vi "CheckImageQuality.vi"(8 "error in (no error)":errorcluster, 11 "Image":T1) -> (0 "error out":errorcluster, 1 "Standard  Variation":sgl, 2 "Mean Value":sgl, 3 "Within Range":bool, 5 "Range":sgl)   [LabVIEW 2017]
uses:
  <vilib>/vision/Image Controls.llb/IMAQ Image.ctl
  <vilib>/vision/NI_Vision_Development_Module.lvlib
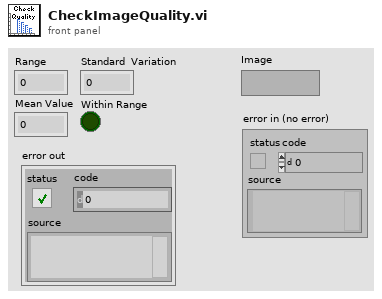
[diagram p1: front panel]
types:
  T1 = typedef "IMAQ Image.ctl" = refnum<image>
  T2 = cluster{"histogram":u32[], "Minimal Value":sgl, "Maximal Value":sgl, "Starting Value":sgl, "Interval Width":sgl, "Mean Value":sgl, "Standard  Variation":sgl, "Area (pixels)":i32}
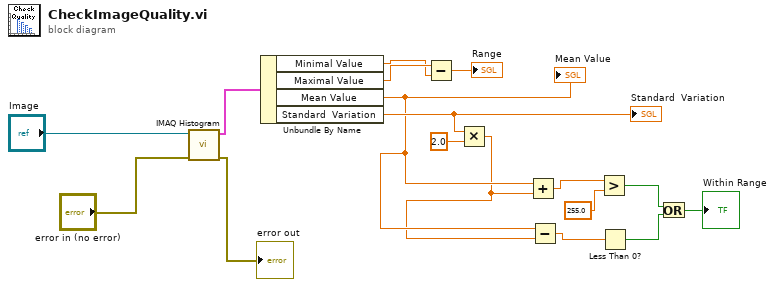
[diagram p0: block diagram]
diagram:
  n1 = call "IMAQ Histogram"("error in (no error)"="error in (no error)", "Image"="Image") -> ("error out"=→"error out":errorcluster, "Histogram Report"=w16:T2)  [unwired: 8 in]
  n2 = Unbundle By Name(w16) -> ("Minimal Value"=w14:sgl, "Maximal Value"=w15:sgl, "Mean Value"=w10:sgl, "Standard  Variation"=w11:sgl)
  "Mean Value" <- w10
  "Standard  Variation" <- w11
  n3 = Subtract(x=w15, y=w14) -> (x-y=→"Range":sgl)
  n4 = Multiply(x=w11, y=2.0) -> (x*y=w9:dbl)
  n5 = Add(x=w10, y=w9) -> (x+y=w4:dbl)
  n6 = Subtract(x=w10, y=w9) -> (x-y=w3:dbl)
  n7 = Greater?(x=w4, y=255.0) -> (0:w7:bool)
  n8 = Less Than 0?(x=w3) -> (x < 0?=w6:bool)
  n9 = Or(x=w7, y=w6) -> (x .or. y?=→"Within Range":bool)
